vi "Write Size Height.vi"(8 "error in (no error)":errorcluster, 10 "Height":u32, 11 "IOName.lvclass in":refnum<class "IOName.lvclass">) -> (0 "error out":errorcluster, 3 "IOName.lvclass out":refnum<class "IOName.lvclass">)   [LabVIEW 2015, in "IOName.lvclass"]
uses:
  IOName.lvclass
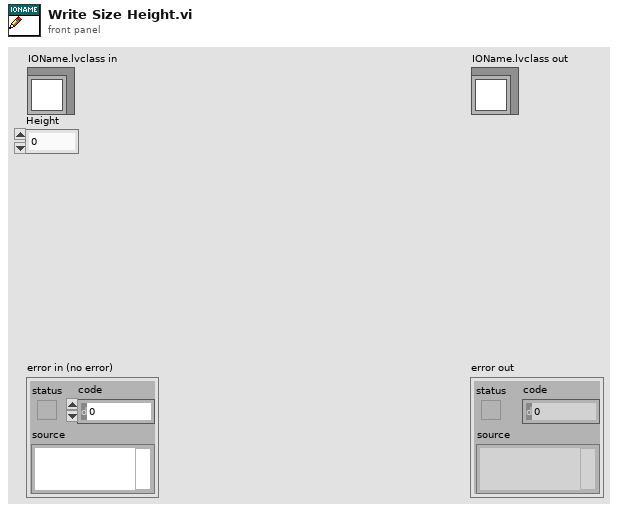
[diagram p1: front panel]
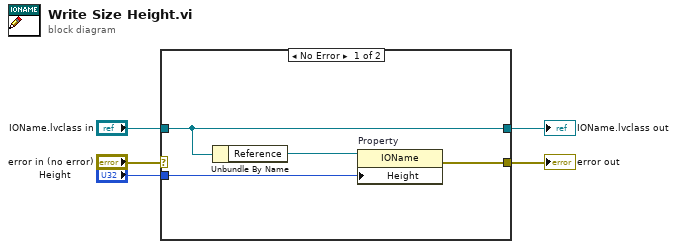
[diagram p0: block diagram]
diagram:
  n1 = case shown="No Error" "error in (no error)" {
    selector: "error in (no error)" -> [_ w11]
    tunnel: [w9 w11] -> w4
    tunnel: [w7 w10] -> w2
    tunnel: "IOName.lvclass in" -> [w7 w10]
    tunnel: "Height" -> [w8 _]
    frame No Error {
      n2 = Unbundle By Name(w7) -> ("Reference"=w6:refnum<vi>)
      n3 = property on="Property" class="IOName"(reference=w6, "Height"=w8) -> (error out=w9:errorcluster)  [unwired: 1 in, 1 out]
    }
    frame Error {
    }
  }
  "error out" <- w4
  "IOName.lvclass out" <- w2
